vi "ArmLimit.vi"(9 "Extend":dbl, 10 "Lift":dbl, 11 "Rotate":dbl) -> (1 "Extend":dbl, 2 "Lift":dbl, 3 "Rotate":dbl)   [LabVIEW 2020]
uses:
  GeneralPurpose/3Dpoint.ctl
  GeneralPurpose/3DCuboid.ctl
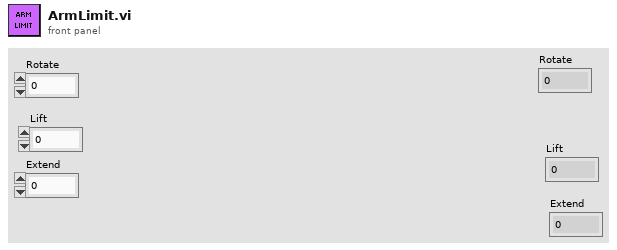
[diagram p1: front panel]
types:
  T1 = typedef "3Dpoint.ctl" = cluster{"X":dbl, "Y":dbl, "Z":dbl}
  T2 = typedef "3DCuboid.ctl" = cluster{"Length(X)":dbl, "Width(Y)":dbl, "Height(Z)":dbl, "OriginPoint":T1}
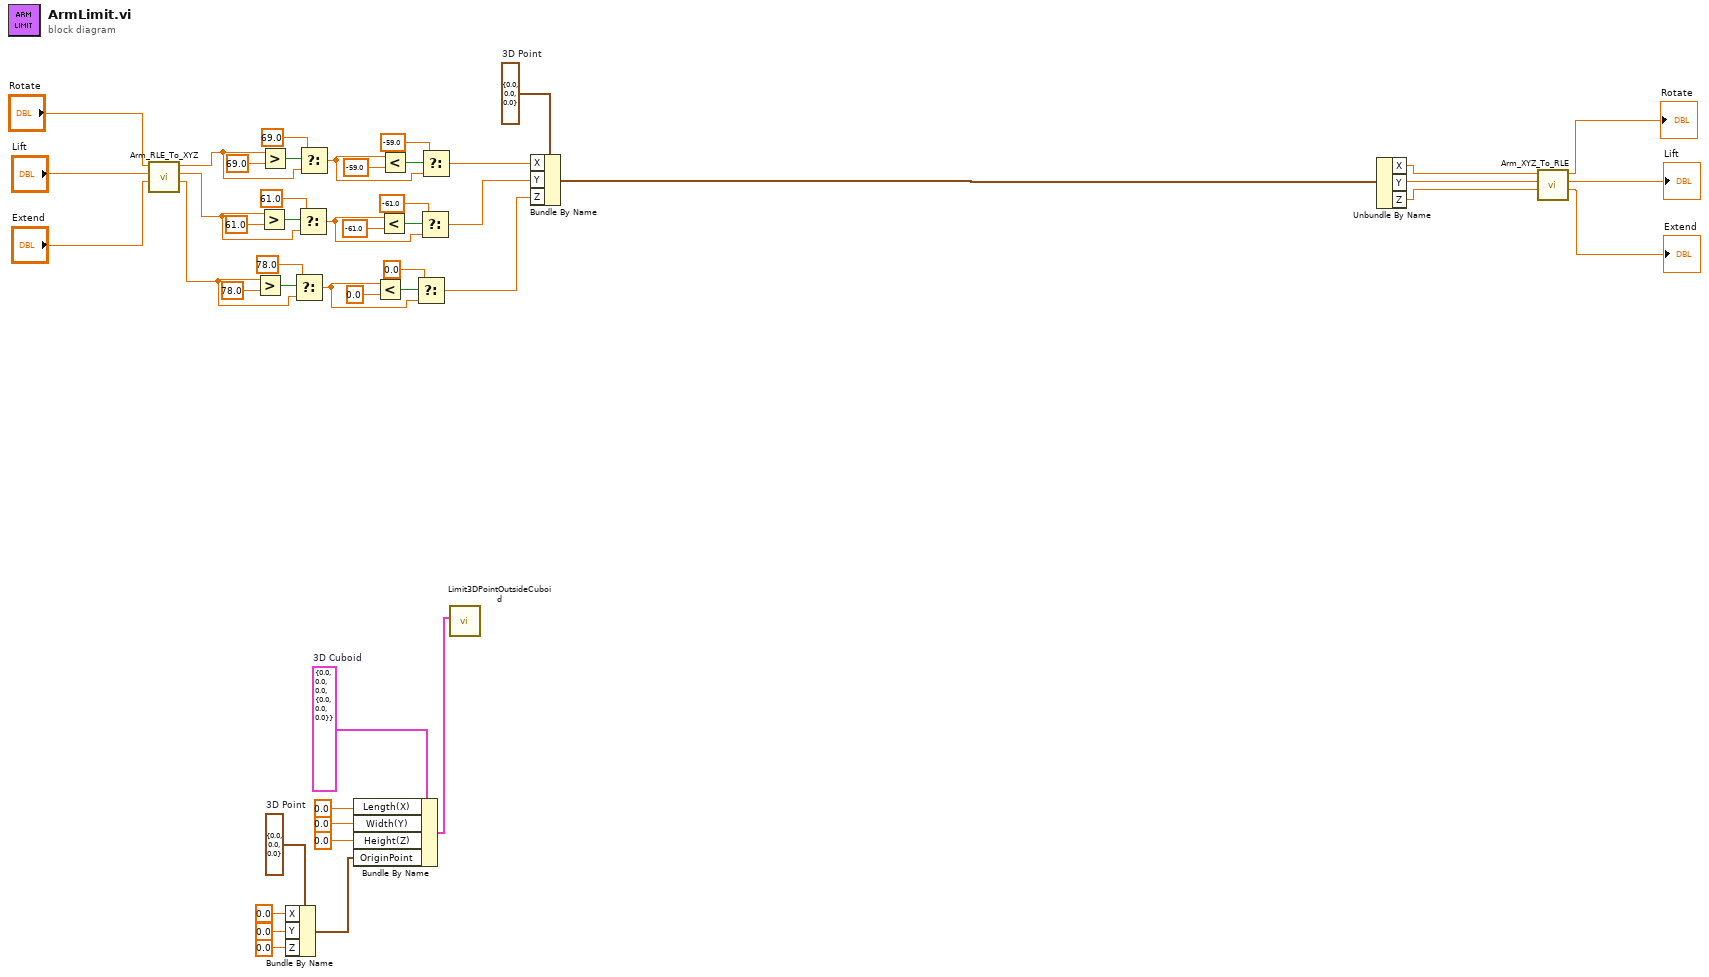
[diagram p0: block diagram]
diagram:
  w37 = T1 {"X"=0.0, "Y"=0.0, "Z"=0.0}  # 3D Point
  w38 = T2 {"Length(X)"=0.0, "Width(Y)"=0.0, "Height(Z)"=0.0, "OriginPoint"={"X"=0.0, "Y"=0.0, "Z"=0.0}}  # 3D Cuboid
  w42 = T1 {"X"=0.0, "Y"=0.0, "Z"=0.0}  # 3D Point
  n1 = call "Arm_RLE_To_XYZ.vi"("Extend"="Extend", "Lift"="Lift", "Rotate"="Rotate") -> ("z"=w3:dbl, "y"=w2:dbl, "x"=w22:dbl)  [unwired: 6 in]
  n2 = Greater?(x=w3, y=78.0) -> (0:w12:bool)
  n3 = Greater?(x=w2, y=61.0) -> (0:w19:bool)
  n4 = Greater?(x=w22, y=69.0) -> (0:w28:bool)
  n5 = Bundle By Name(cluster=w37, "X"=0.0, "Y"=0.0, "Z"=0.0) -> (w36:T1)
  n6 = Select(t=78.0, s=w12, f=w3) -> (s? t:f=w7:dbl)
  n7 = Select(t=61.0, s=w19, f=w2) -> (s? t:f=w14:dbl)
  n8 = Select(t=69.0, s=w28, f=w22) -> (s? t:f=w23:dbl)
  n9 = Bundle By Name(cluster=w38, "Length(X)"=0.0, "Width(Y)"=0.0, "Height(Z)"=0.0, "OriginPoint"=w36) -> (w29:T2)
  n10 = Less?(x=w7, y=0.0) -> (x < y?=w11:bool)
  n11 = Less?(x=w14, y=-61.0) -> (x < y?=w18:bool)
  n12 = Less?(x=w23, y=-59.0) -> (x < y?=w27:bool)
  n13 = Select(t=0.0, s=w11, f=w7) -> (s? t:f=w4:dbl)
  n14 = Select(t=-61.0, s=w18, f=w14) -> (s? t:f=w5:dbl)
  n15 = Select(t=-59.0, s=w27, f=w23) -> (s? t:f=w20:dbl)
  n16 = call "Limit3DPointOutsideCuboid.vi"("3D Cuboid"=w29) -> ()  [unwired: 10 in, 1 out]
  n17 = Bundle By Name(cluster=w42, "X"=w20, "Y"=w5, "Z"=w4) -> (w1:T1)
  n18 = Unbundle By Name(w1) -> ("X"=w41:dbl, "Y"=w40:dbl, "Z"=w39:dbl)
  n19 = call "Arm_XYZ_To_RLE.vi"("Z"=w39, "Y"=w40, "X"=w41) -> ("Extend"=→"Extend":dbl, "Lift"=→"Lift":dbl, "Rotate"=→"Rotate":dbl)  [unwired: 6 in]
